vi "Pickup Down State.vi"(11 "Trigger":bool) -> ()   [LabVIEW 2013]
uses:
  <vilib>/Rock Robotics/WPI/Solenoid/Deprecated/WPI_SolenoidSetBool.vi
panel:
  out "Wait":bool
  out "Boolean":bool
  out "Elapsed Time (s) 2":dbl caption="Elapsed Time (s)"
  out "Arm Down":bool
  out "Clamp Open":bool
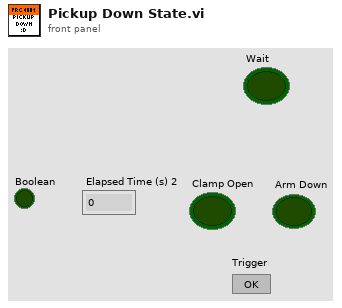
[diagram p1: front panel]
types:
  T1 = typedef "WPI_SolenoidDevRef.ctl" = cluster{"DevStatus":errorcluster, "Solenoid Module":T2, "Forward Solenoid Channel":T3, "Reverse Solenoid Channel":T3}
  T2 = typedef "FPGA_TypedefSolenoidModule.ctl" = enum16{"Solenoid Module 1", "Solenoid Module 2"}
  T3 = typedef "WPI_SolenoidChannel.ctl" = enum8{"Solenoid 1", "Solenoid 2", "Solenoid 3", "Solenoid 4", "Solenoid 5", "Solenoid 6", "Solenoid 7", "Solenoid 8", "Invalid"}
  T4 = typedef "WPI_MotorControlDeviceRef.ctl" = cluster{"DeviceStatus":errorcluster, "Type":enum16{"PWM", "CAN"}, "PWM":cluster{"Digital Module":T5, "PWM Channel":T6, "DeadBand":T7}, "CAN":cluster{"Device Number":u8, "Control Mode":T8, "Semaphore":T9, "Max Vout":dbl}, "Invert":bool, "TransformRef":T10, "InvTransformRef":T10}
  T5 = typedef "FPGA_TypedefDigitalModule.ctl" = enum16{"Digital Module 1", "Digital Module 2"}
  T6 = typedef "FPGA_DIOPWMChannel.ctl" = enum8{"PWM 1", "PWM 2", "PWM 3", "PWM 4", "PWM 5", "PWM 6", "PWM 7", "PWM 8", "PWM 9", "PWM 10", "Invalid"}
  T7 = typedef "WPI_PWMDeadband.ctl" = cluster{"Name":string, "maxPositivePwm":i32, "minPositivePwm":i32, "centerPwm":i32, "maxNegativePwm":i32, "minNegativePwm":i32, "angularRange":u16}
  T8 = typedef "WPI_CANJaguar_ControlMode.ctl" = enum8{"Percent VBus", "Current", "Speed", "Position", "Voltage"}
  T9 = typedef "Semaphore RefNum" = refnum<k1>
  T10 = typedef "WPI_PWMTransform_ConPane.ctl" = refnum<vi>
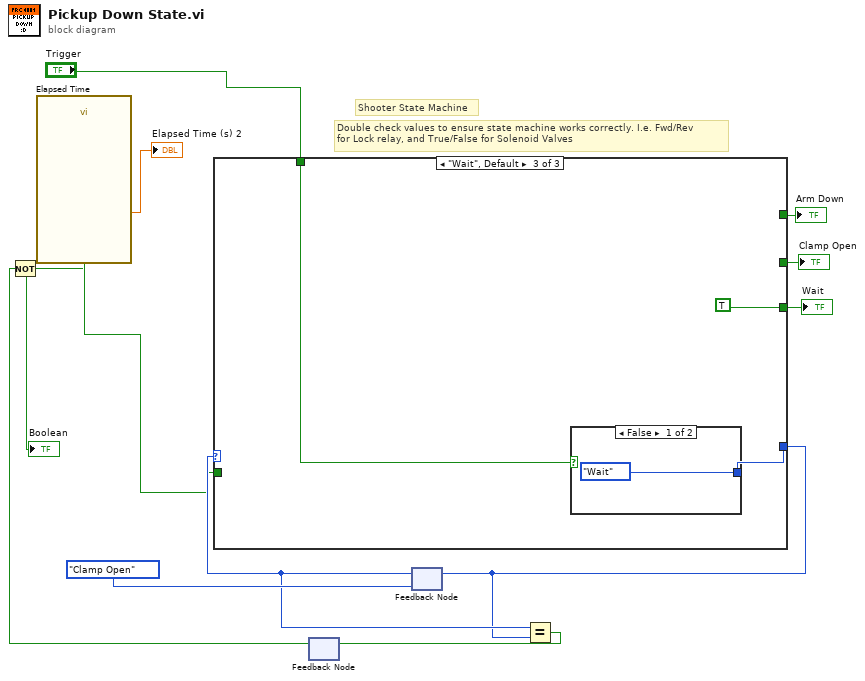
[diagram p0: block diagram]
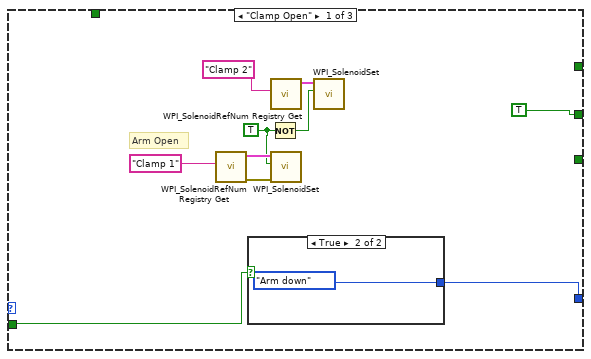
[diagram p2: hidden frame]
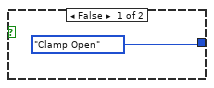
[diagram p3: hidden frame]
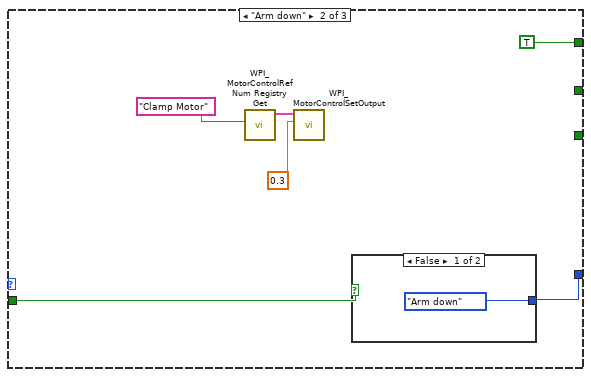
[diagram p4: hidden frame]
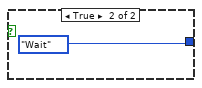
[diagram p5: hidden frame]
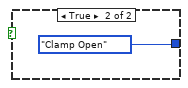
[diagram p6: hidden frame]
diagram:
  # "Double check values to ensure state machine works correctly. I.e. Fwd/Rev\nfor Lock relay, and True/False for Solenoid Valves"
  # "Shooter State Machine"
  n1 = feedback #1() -> (w5:bool)  [unwired: 1 in]
  n2 = Not(x=w5) -> (.not. x?=w3:bool)
  "Boolean" <- w3
  n3 = call "Elapsed Time"("Reset"=w3) -> ("Elapsed Time (s)"=→"Elapsed Time (s) 2":dbl, "Time has Elapsed"=w4:bool)  [unwired: 11 in, 6 out]
  n4 = feedback #2(enum16{"Clamp Open", "Arm down", "Wait"}."Clamp Open") -> (w9:enum16{"Clamp Open", "Arm down", "Wait"})
  n5 = case shown="\"Wait\", Default" w9 {
    tunnel: [w22 w30 w35] -> w8
    tunnel: [TRUE ("State 0") _ _] -> w11
    tunnel: [_ TRUE _] -> w10
    tunnel: w4 -> [w13 w28 _]
    tunnel: "Trigger" -> [_ _ w33]
    tunnel: [_ _ TRUE] -> w1
    frame "Clamp Open" {
      w14 = TRUE ("x")
      # "Arm Open"
      n6 = call <vilib>:"WPI_SolenoidRefNum Registry Get.vi"("refnum name"="Clamp 1") -> ("error out"=w18:errorcluster, "SolenoidDevRef"=w19:T1)  [unwired: 9 in]
      n7 = case shown="True" w13 {
        tunnel: [enum16{"Clamp Open", "Arm down", "Wait"}."Clamp Open" enum16{"Clamp Open", "Arm down", "Wait"}."Arm down"] -> w22
        frame False {
        }
        frame True {
        }
      }
      n8 = Not(x=w14) -> (.not. x?=w15:bool)
      n9 = call <vilib>:"WPI_SolenoidRefNum Registry Get.vi"("refnum name"="Clamp 2") -> ("SolenoidDevRef"=w17:T1)  [unwired: 9 in, 1 out]
      n10 = call-poly <vilib>:"WPI_SolenoidSet.vi"("error in (no error)"=w18, "Value"=w14, "SolenoidDevRef"=w19) -> ()  [unwired: 7 in, 2 out]
      n11 = call-poly <vilib>:"WPI_SolenoidSet.vi"("Value"=w15, "SolenoidDevRef"=w17) -> ()  [unwired: 8 in, 2 out]
    }
    frame "Arm down" {
      n12 = call <vilib>:"WPI_MotorControlRefNum Registry Get.vi"("refnum name"="Clamp Motor") -> ("MotorControlDevRef"=w26:T4)  [unwired: 9 in, 1 out]
      n13 = call <vilib>:"WPI_MotorControlSetOutput.vi"("Output"=0.3, "MotorControlDevRef"=w26) -> ()  [unwired: 7 in, 3 out]
      n14 = case shown="False" w28 {
        tunnel: [enum16{"Clamp Open", "Arm down", "Wait"}."Arm down" enum16{"Clamp Open", "Arm down", "Wait"}."Wait"] -> w30
        frame False {
        }
        frame True {
        }
      }
    }
    frame "Wait", Default {
      n15 = case shown="False" w33 {
        tunnel: [enum16{"Clamp Open", "Arm down", "Wait"}."Wait" enum16{"Clamp Open", "Arm down", "Wait"}."Clamp Open"] -> w35
        frame False {
        }
        frame True {
        }
      }
    }
  }
  "Clamp Open" <- w11
  "Arm Down" <- w10
  "Wait" <- w1
  n16 = feedback-in #2(w8) -> ()
  n17 = Equal?(x=w9, y=w8) -> (x = y?=w6:bool)
  n18 = feedback-in #1(w6) -> ()
